vi "LCR_Readout.vi"(8 "error in (no error)":errorcluster, 10 "Frequency in Hz":i32, 11 "WK6440B in":refnum<class "WK6440B.lvclass">) -> (0 "error out":errorcluster, 1 "Resistance in Ohm":dbl, 2 "Capacitance in pF":dbl, 3 "WK6440B out":refnum<class "WK6440B.lvclass">)   [LabVIEW 2018, in "WK6440B.lvclass"]
uses:
  WK6440B.lvclass
  C:/Users/Graham Greig/Desktop/itk-strip-sensor-qc-master/itk-strip-sensor-qc-master/InstrControl/InstrControl.lvclass
  InstrControl.lvclass
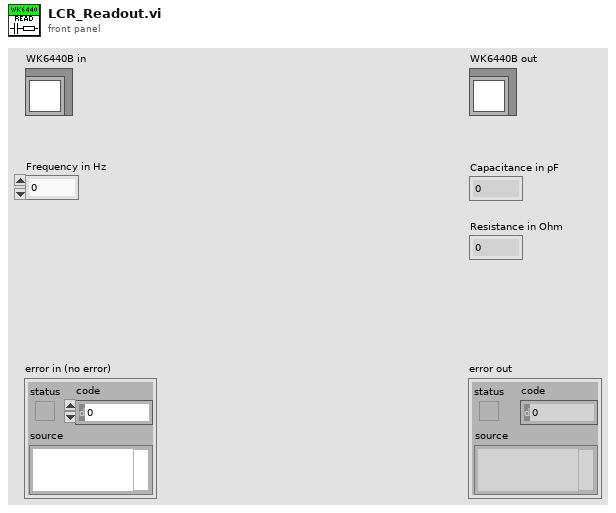
[diagram p1: front panel]
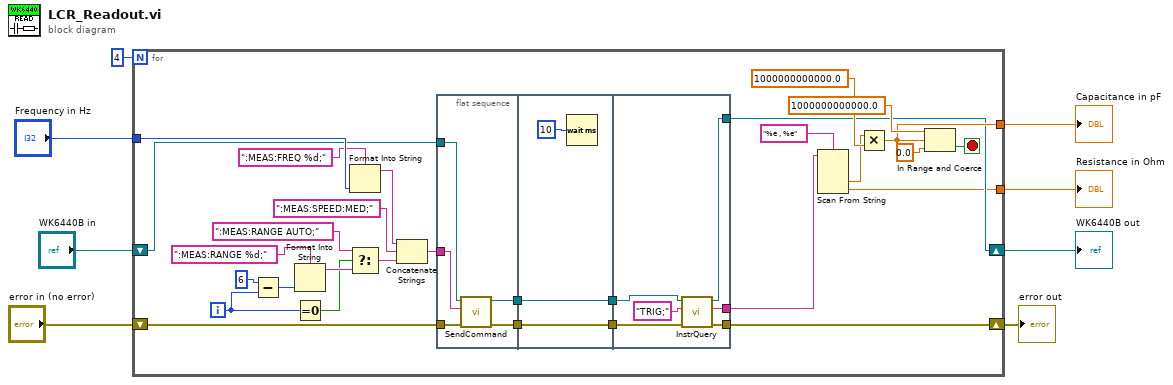
[diagram p0: block diagram]
diagram:
  n1 = for {
    N: 4 -> [_]
    tunnel: [w9] -> w4
    tunnel: [w35] -> w5
    tunnel: "Frequency in Hz" -> [w32]
    shift-right: [w10] -> w1
    shift-left: "WK6440B in" -> [w17]
    shift-right: [w15] -> w6
    shift-left: "error in (no error)" -> [w31]
    i -> [w34]
    stop <- w33 stop-if-true
    n2 = Subtract(x=6, y=w34) -> (x-y=w21:i32)
    n3 = Format Into String(format string=":MEAS:RANGE %d;", w21) -> (resulting string=w24:string)  [unwired: 2 in, 1 out]
    n4 = Equal To 0?(x=w34) -> (x = 0?=w23:bool)
    n5 = Format Into String(format string=":MEAS:FREQ %d;", w32) -> (resulting string=w30:string)  [unwired: 2 in, 1 out]
    n6 = Select(t=":MEAS:RANGE AUTO;", s=w23, f=w24) -> (s? t:f=w27:string)
    n7 = Concatenate Strings(w30, ":MEAS:SPEED:MED;", w27) -> (w38:string)
    n8 = flat-sequence {
      tunnel: w38 -> [w41]
      tunnel: w31 -> [w43]
      tunnel: w17 -> [w39]
      tunnel: [w42] -> w14
      tunnel: [w40] -> w12
      tunnel: w14 -> [w45]
      tunnel: [w45] -> w13
      tunnel: w12 -> [w44]
      tunnel: [w44] -> w11
      tunnel: [w51] -> w15
      tunnel: [w50] -> w16
      tunnel: w13 -> [w52]
      tunnel: w11 -> [w48]
      tunnel: [w47] -> w10
      frame #0 {
        n9 = call "SendCommand.vi"("error in (no error)"=w43, "Command string"=w41, "InstControl in"=w39) -> ("error out"=w42:errorcluster, "InstControl out"=w40:refnum<class "WK6440B.lvclass">)  [unwired: 7 in]
      }
      frame #1 {
        n10 = Wait (ms)(milliseconds to wait=10) -> ()  [unwired: 1 out]
      }
      frame #2 {
        n11 = call-dynamic "InstrQuery.vi"("error in (no error)"=w52, "Command string"="TRIG;", "InstControl in"=w48) -> ("error out"=w51:errorcluster, "Instrument response"=w50:string, "InstControl out"=w47:refnum<class "WK6440B.lvclass">)  [unwired: 6 in]
      }
    }
    n12 = Scan From String(format string="%e , %e", input string=w16) -> (output 1=w18:dbl, output 2=w9:dbl)  [unwired: 4 in, 3 out]
    n13 = Multiply(x=w18, y=1000000000000.0) -> (x*y=w35:dbl)
    n14 = In Range and Coerce(upper limit=1000000000000.0 ("y"), x=w35, lower limit=0.0) -> (In Range?=w33:bool)  [unwired: 1 out]
  }
  "error out" <- w6
  "WK6440B out" <- w1
  "Capacitance in pF" <- w5
  "Resistance in Ohm" <- w4
